vi "Set_Sequence_Text_Argument.vi"(2 "Text":string, 3 "Argument":string, 4 "Index":i32, 5 "Input Sequence":cluster{string, string[], dbl[], dbl}[](array[cluster])) -> (0 "Argument String":string, 1 "Output Sequence":cluster{string, string[], dbl[], dbl}[](array[cluster]))   [LabVIEW 2011]
doc: "This VI sets the value of a textual argument in the context of the sequence. It is identical to Set_Text_Argument.vi but instead of operating on an individual event directly, it operates on a certain event in a sequence determined by the \"Index\" parameter."
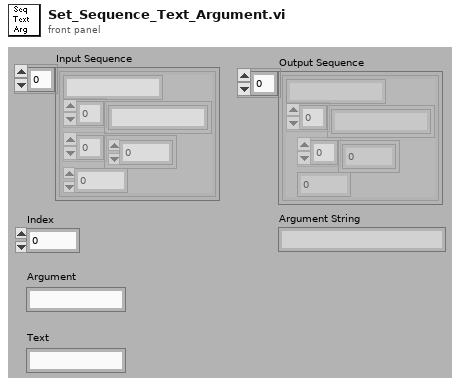
[diagram p1: front panel]
types:
  T1 = cluster{string, "Argument List Out":string[], dbl[], dbl}
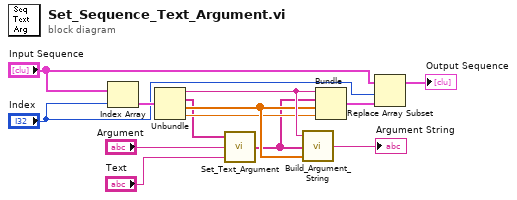
[diagram p0: block diagram]
diagram:
  n1 = Index Array(array="Input Sequence", index="Index") -> (element=w13:cluster{string, string[], dbl[], dbl})
  n2 = Unbundle(w13) -> (w11:string, w3:string[], w10:dbl[], w9:dbl)
  n3 = call "Set_Text_Argument.vi"("Text"="Text", "Argument"="Argument", "Argument List In"=w3) -> ("Argument List Out"=w4:string[])
  n4 = call "Build_Argument_String.vi"("Flow Array"=w10, "Argument List"=w4, "Command"=w11) -> ("Argument String"=→"Argument String":string)
  n5 = Bundle(w11, "Argument List Out"=w4, w10, w9) -> (w8:T1)  [unwired: 1 out]
  n6 = Replace Array Subset(array="Input Sequence", new element=w8, index="Index") -> (→"Output Sequence":cluster{string, string[], dbl[], dbl}[])
